vi "destroy.vi"(8 "error in (no error)":errorcluster, 11 "tree (dvr)":refnum<data-value>) -> (0 "error []":errorcluster[](array[cluster]))   [LabVIEW 2015, in "binary_tree.lvlib"]
uses:
  binary_tree.lvlib
  _Controls/tree.ctl
  _Controls/node_key.ctl
  _Controls/node_data.ctl
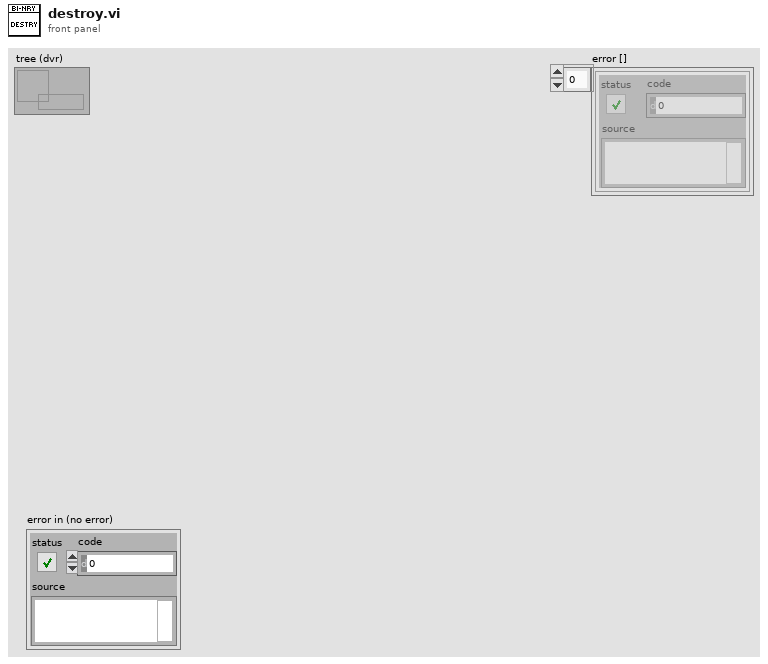
[diagram p1: front panel]
types:
  T1 = typedef "binary_tree.lvlib/tree.ctl" = cluster{"key":T2, "data":T3, "node_dvr (left)":variant, "node_dvr (right)":variant}
  T2 = typedef "binary_tree.lvlib/node_key.ctl" = cluster{dbl}
  T3 = typedef "binary_tree.lvlib/node_data.ctl" = cluster{dbl}
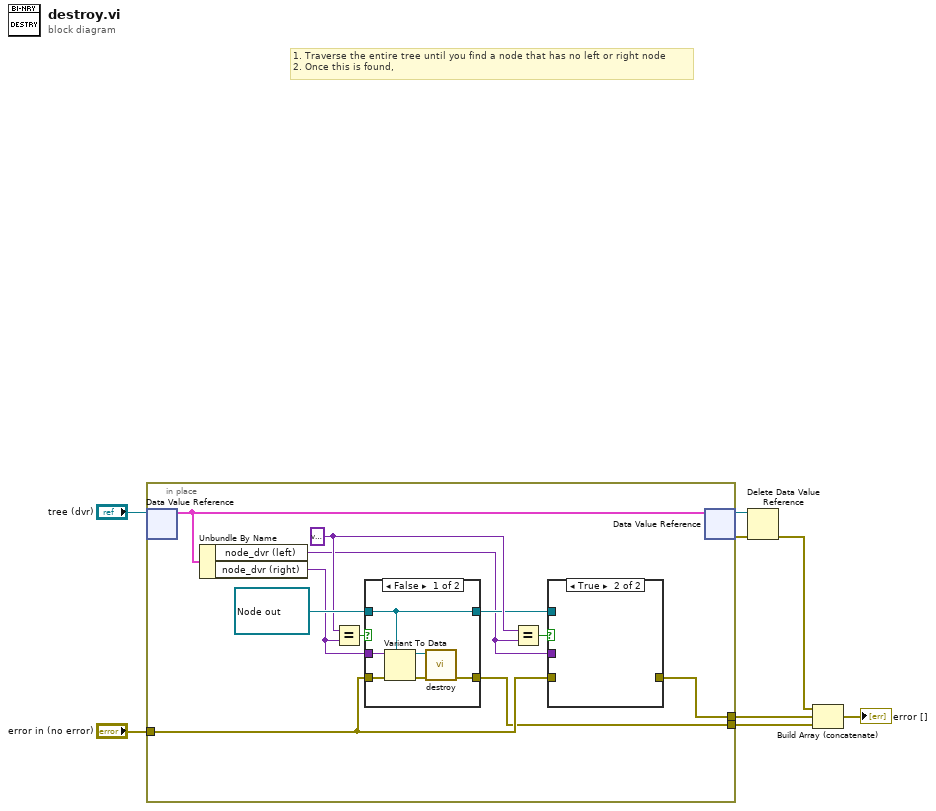
[diagram p0: block diagram]
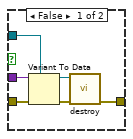
[diagram p2: hidden frame]
diagram:
  # "1. Traverse the entire tree until you find a node that has no left or right node\n2. Once this is found,"
  n1 = in-place {
    in-place-border: [w13] -> w7
    in-place-border: "error in (no error)" -> [w10]
    in-place-border: [w9] -> w1
    w16 = variant ("Left")
    n2 = in-place-dvr #1("tree (dvr)") -> (w19:T1)  [unwired: 1 out]
    n3 = Unbundle By Name(w19) -> ("node_dvr (left)"=w11:variant, "node_dvr (right)"=w17:variant)
    n4 = Equal?(x=w16, y=w17) -> (x = y?=w15:bool)
    n5 = case shown="False" w15 {
      tunnel: w17 -> [w31 _]
      tunnel: [w29 _] -> w9
      tunnel: refnum<data-value> refnum ("tree (dvr)") -> [w27 w32]
      tunnel: [w27 w32] -> w12
      tunnel: w10 -> [w26 _]
      frame False {
        n6 = Variant To Data(error in=w26, type=w27, Variant=w31) -> (data=w28:refnum<data-value>, error out=w30:errorcluster)
        n7 = call "destroy.vi"("error in (no error)"=w30, "tree (dvr)"=w28) -> ("error []"=w29:errorcluster[])  [unwired: 9 in]
      }
      frame True {
      }
    }
    n8 = Equal?(x=w16, y=w11) -> (x = y?=w14:bool)
    n9 = case shown="True" w14 {
      tunnel: w10 -> [w25 _]
      tunnel: w11 -> [w24 _]
      tunnel: [w22 _] -> w13
      tunnel: w12 -> [w21 _]
      frame False {
        n10 = Variant To Data(error in=w25, type=w21, Variant=w24) -> (data=w20:refnum<data-value>, error out=w23:errorcluster)
        n11 = call "destroy.vi"("error in (no error)"=w23, "tree (dvr)"=w20) -> ("error []"=w22:errorcluster[])  [unwired: 9 in]
      }
      frame True {
      }
    }
    n12 = in-place-dvr #1(w19) -> (w6:refnum<data-value>, w5:errorcluster)
  }
  n13 = Delete Data Value Reference(data value reference=w6, error in=w5) -> (error out=w4:errorcluster)  [unwired: 1 out]
  n14 = Build Array (concatenate)(w4, w7, w1) -> (→"error []":errorcluster[])
